vi "main_camera_acquisition.vi"() -> ()   [LabVIEW 2009]
uses:
  <vilib>/userdefined/High Color/IMAQdx.ctl
  <vilib>/vision/Image Controls.llb/IMAQ Image.ctl
  <vilib>/vision/driver/IMAQdx.llb/IMAQdx Buffer Number Mode.ctl
  <vilib>/vision/driver/NI_Vision_Acquisition_Software.lvlib
  Program Files (x86)/National Instruments/LabVIEW 2009/resource/objmgr/imaqdx.rc
panel:
  in  "Video Mode":u32=2
  out "ROI table":string[](array[string])=["Breite [px]", "Höhe [px]", "X-Offset [px]", "Y-Offset [px]"]
  in  "Vollbild":bool
  in  "Y Offset (px)":u32
  in  "X Offset (px)":u32
  in  "Image Height (px)":u32=480
  in  "Image Width (px)":u32=640
  in  "ROI":i32[](array[numeric])=[640, 480, 0, 0]
  in  "Shutter time (ms)":u16(ring)=3 items=["1000", "500", "200", "100", "50", "20", "10", "1"]
  out "Buffer Overrun":bool
  out "Buffer Number":u32
  out "Frame Rate (FPS)":dbl format="%#_3g"
  out "Image Memory":T1
  in  "Buffer Interval":u32=1
  out "Ereignis: FrameDone?":refnum<event-registration>
  out "Camera eingeschaltet":bool
  in  "Kamera ON/OFF":bool
  in  "Stopp":bool
  in  "Detektionskamera":T2="cam0"
  out "Error Out":errorcluster
  out "Image Display":T1(plugin-control)
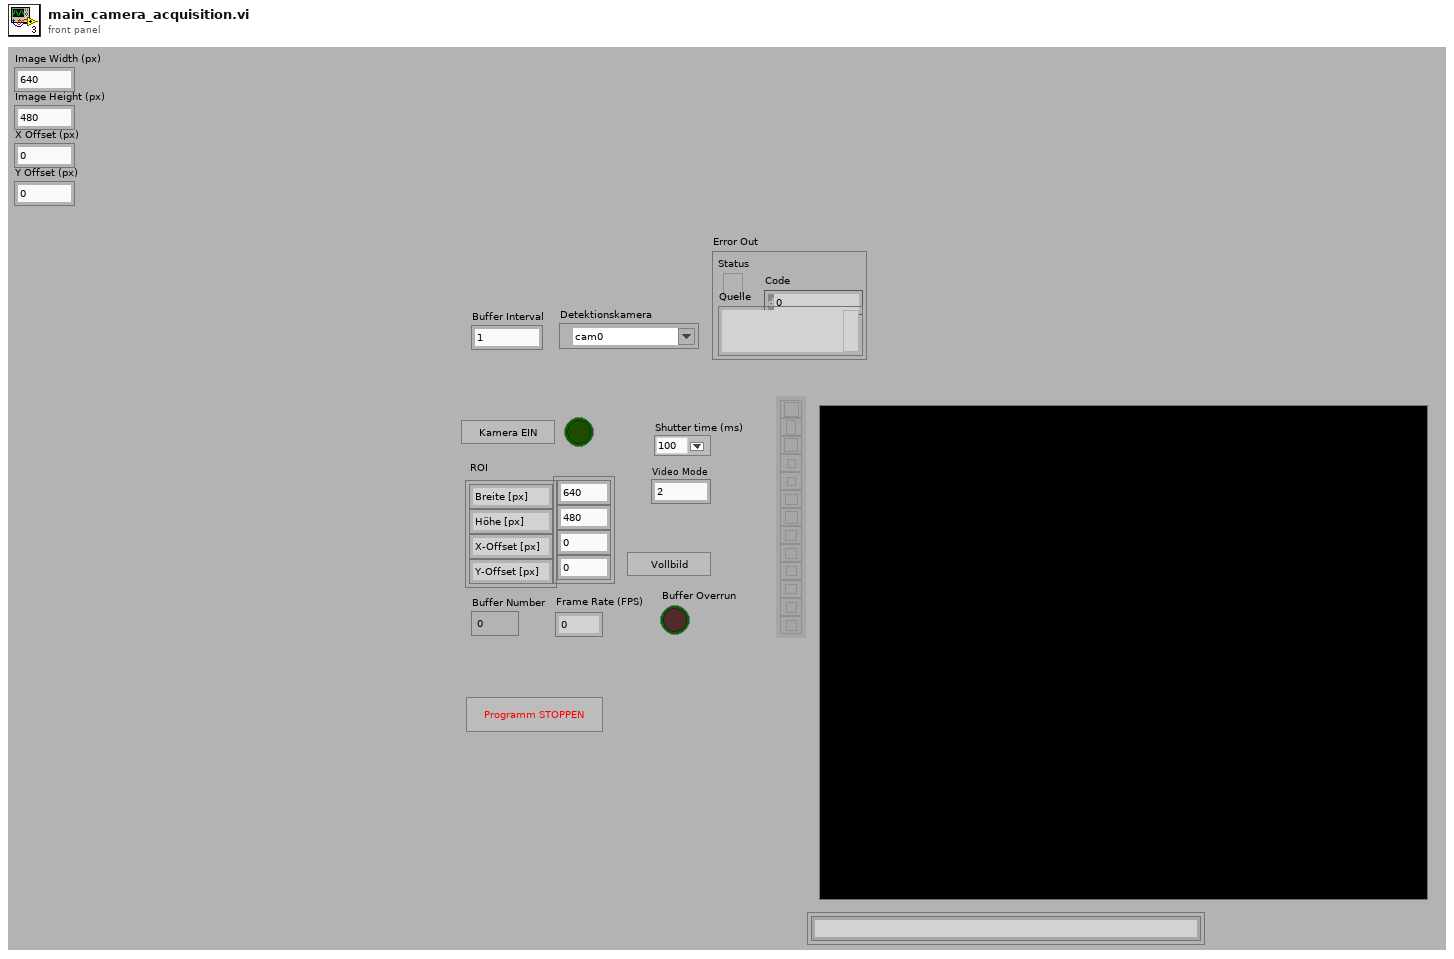
[diagram p1: front panel]
types:
  T1 = typedef "IMAQ Image.ctl" = refnum<image>
  T2 = typedef "IMAQdx.ctl" = refnum<k21>
  T3 = typedef "NI_Vision_Acquisition_Software.lvlib/IMAQdx Buffer Number Mode.ctl" = enum32{"Next", "Last", "Buffer Number"}
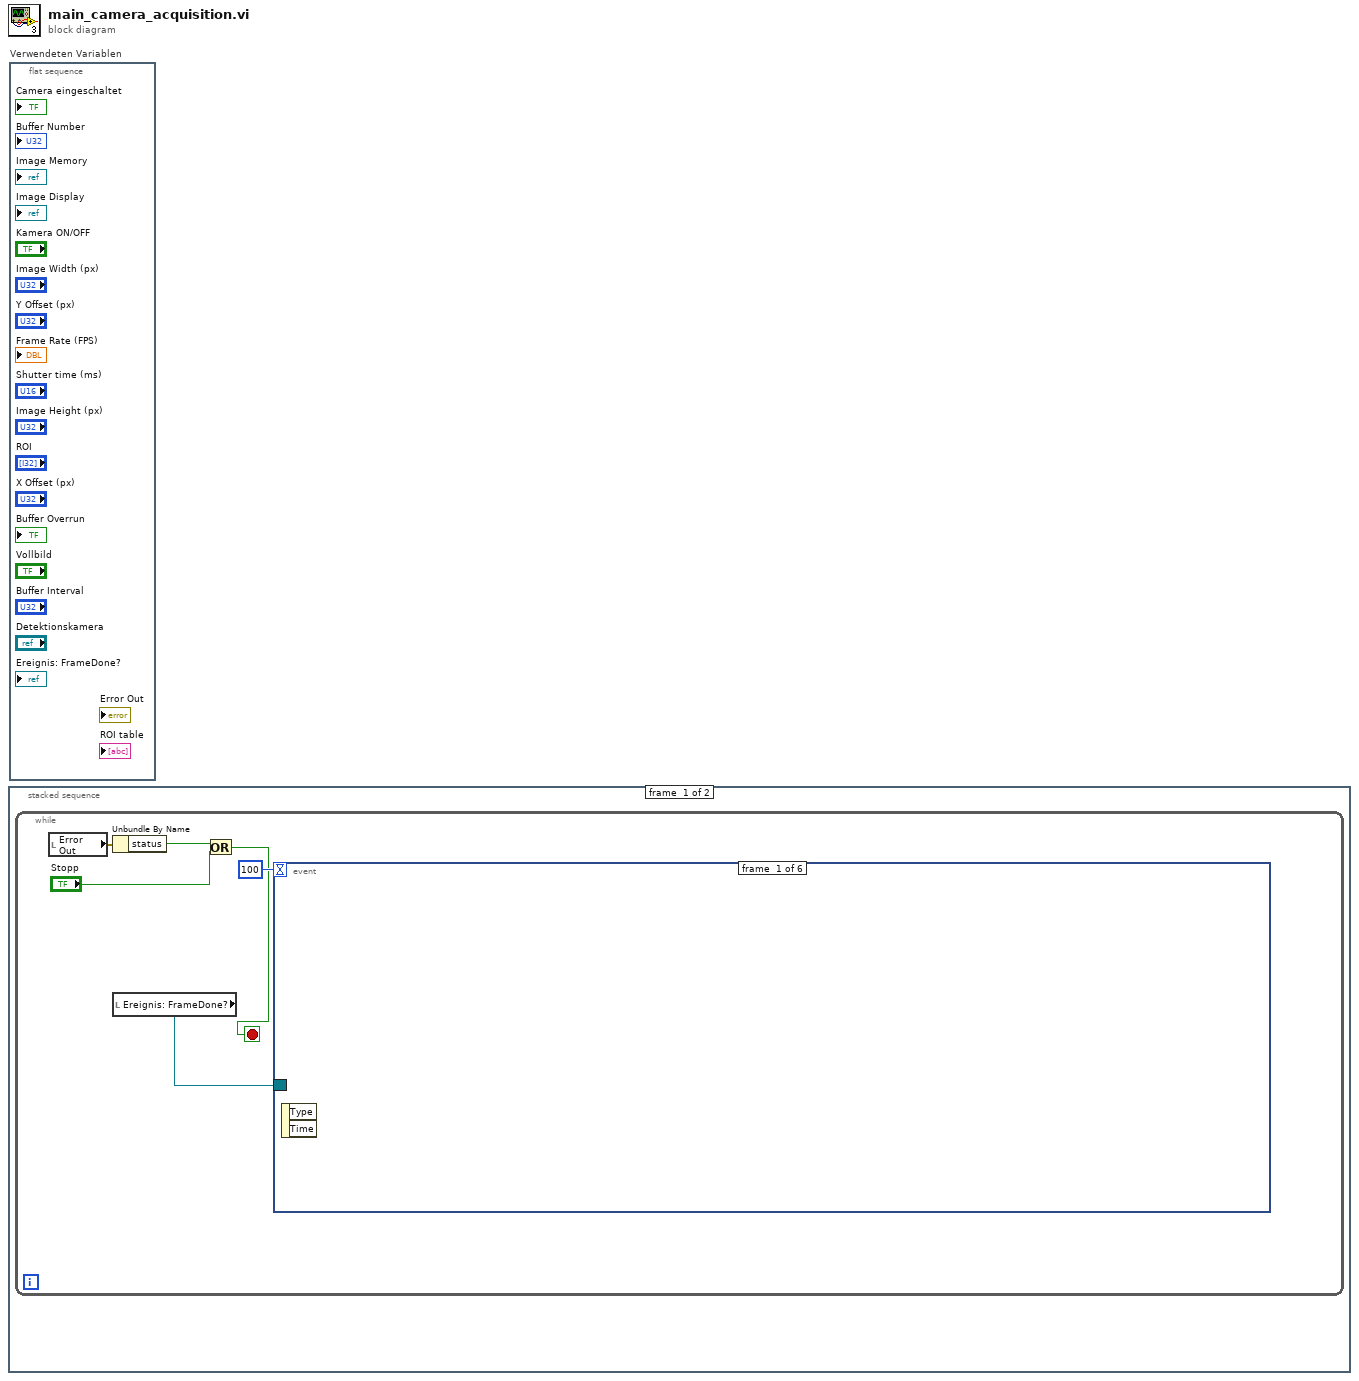
[diagram p0: block diagram]
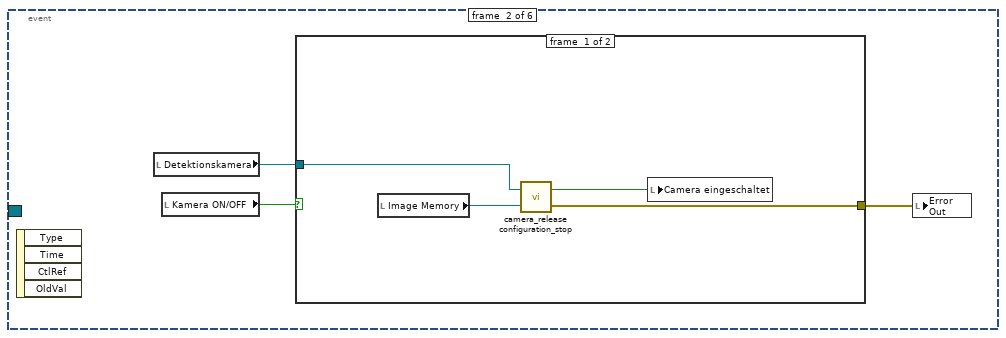
[diagram p2: hidden frame]
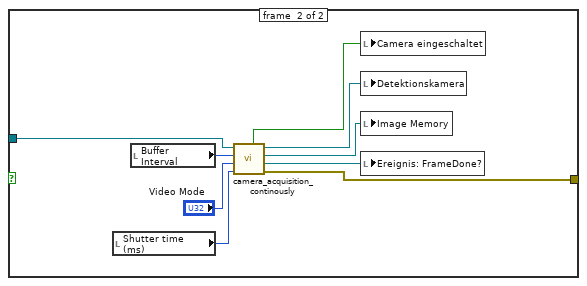
[diagram p3: hidden frame]
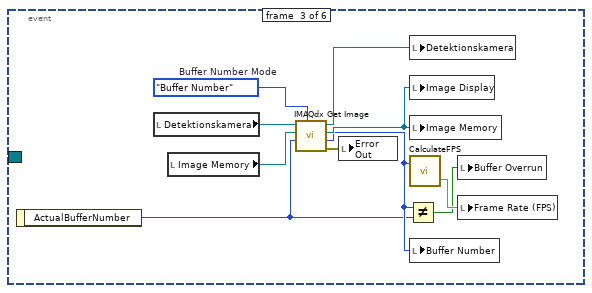
[diagram p4: hidden frame]
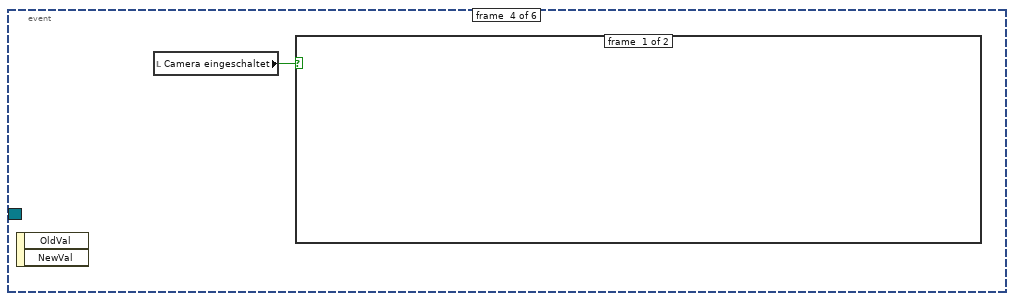
[diagram p5: hidden frame]
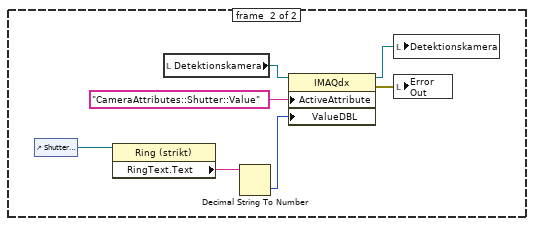
[diagram p6: hidden frame]
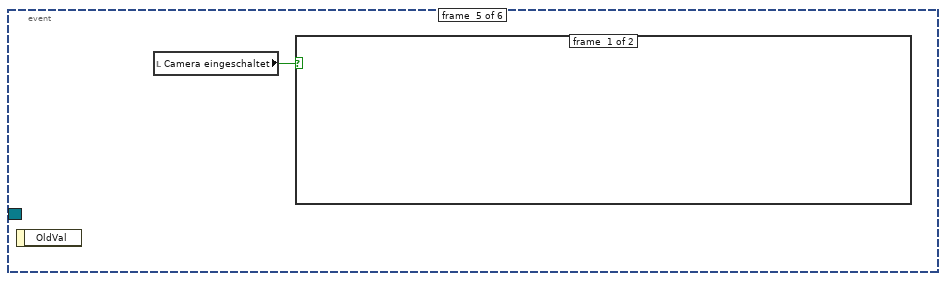
[diagram p7: hidden frame]
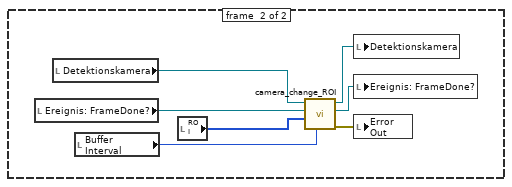
[diagram p8: hidden frame]
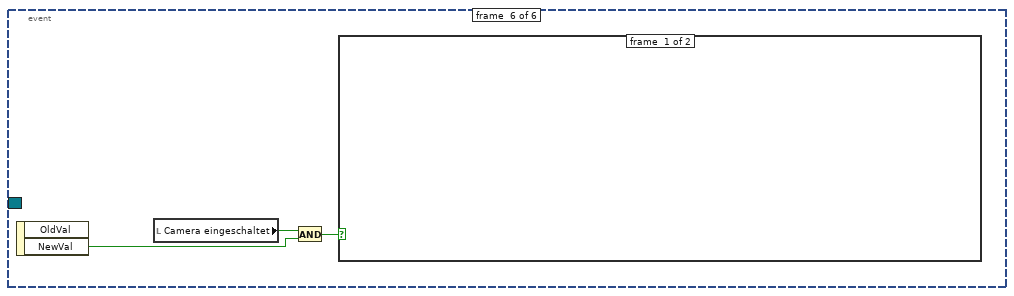
[diagram p9: hidden frame]
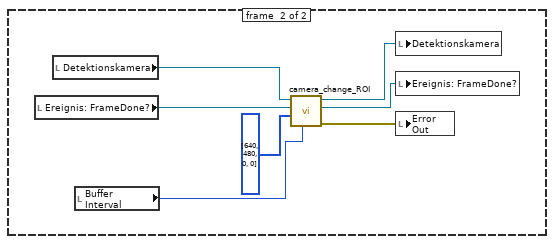
[diagram p10: hidden frame]
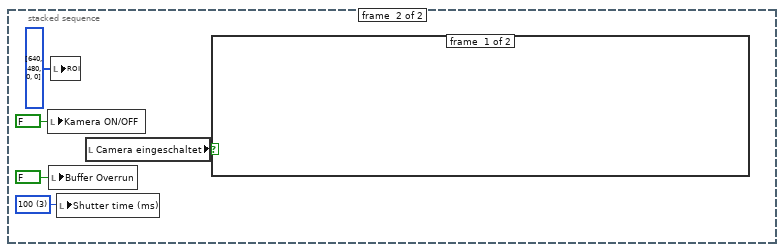
[diagram p11: hidden frame]
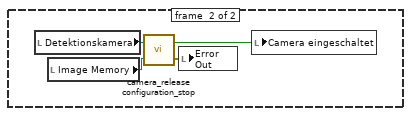
[diagram p12: hidden frame]
diagram:
  n1 = stacked-sequence {
    frame #0 {
      n2 = while {
        stop <- w3 stop-if-true
        n3 = local read "Error Out"() -> (w2:errorcluster)
        n4 = Unbundle By Name(w2) -> ("status"=w1:bool)
        n5 = local read "Ereignis: FrameDone?"() -> (w5:refnum<event-registration>)
        n6 = Or(x=w1, y="Stopp") -> (x .or. y?=w3:bool)
        n7 = event shown="[1] \"Kamera ON/OFF\": Wertänderung" {
          selector: w5 -> [_ _ _ _ _ _]
          dyn-events: _ -> [_ _ _ _ _ _]
          timeout: 100 -> [_ _ _ _ _ _]
          event #0 {
            n8 = event-data() -> ()  [unwired: 1 in, 2 out]
          }
          event #1 {
            n9 = event-data() -> ()  [unwired: 1 in, 4 out]
            n10 = local read "Detektionskamera"() -> (w8:T2)
            n11 = local read "Kamera ON/OFF"() -> (w9:bool)
            n12 = case shown="True" w9 {
              tunnel: w8 -> [w10 w17]
              tunnel: [w13 w18] -> w7
              frame #0 {
                n13 = local read "Image Memory"() -> (w11:T1)
                n14 = call "camera_release configuration_stop.vi"("Image Memory"=w11, "Detektionskamera"=w10) -> ("error out"=w13:errorcluster, "status"=w12:bool)
                n15 = local write "Camera eingeschaltet"(w12) -> ()
              }
              frame #1 {
                n16 = local read "Shutter time (ms)"() -> (w14:u16)
                n17 = local read "Buffer Interval"() -> (w16:u32)
                n18 = call "camera_acquisition_continously.vi"("Detektionskamera"=w17, "BufferInterval"=w16, "Video Mode"="Video Mode", "Shutter time (ms)"=w14) -> ("Kamera eingeschaltet?"=w22:bool, "Detektionskamera"=w21:T2, "Image Memory"=w20:T1, "Ereignis: FrameDone?"=w19:refnum<event-registration>, "error out"=w18:errorcluster)
                n19 = local write "Camera eingeschaltet"(w22) -> ()
                n20 = local write "Detektionskamera"(w21) -> ()
                n21 = local write "Image Memory"(w20) -> ()
                n22 = local write "Ereignis: FrameDone?"(w19) -> ()
              }
            }
            n23 = local write "Error Out"(w7) -> ()
          }
          event #2 {
            w32 = IMAQdx_Buffer_Number_Mode."Buffer Number"  # Buffer Number Mode
            n24 = event-data() -> ("ActualBufferNumber"=w24:u32)  [unwired: 1 in]
            n25 = local read "Detektionskamera"() -> (w30:T2)
            n26 = local read "Image Memory"() -> (w29:T1)
            n27 = call <vilib>:"IMAQdx Get Image.vi"("Buffer Number Mode (Next)"=w32, "Buffer Number In"=w24, "Image In"=w29, "Session In"=w30) -> ("error out"=w31:errorcluster, "Buffer Number Out"=w25:u32, "Image Out"=w27:T1, "Session Out"=w26:T2)  [unwired: 1 in, 3 out]
            n28 = local write "Error Out"(w31) -> ()
            n29 = Not Equal?(x=w25, y=w24) -> (x != y?=w23:bool)
            n30 = local write "Detektionskamera"(w26) -> ()
            n31 = local write "Image Display"(w27) -> ()
            n32 = local write "Image Memory"(w27) -> ()
            n33 = call "CalculateFPS.vi"("buffer number"=w25) -> ("processed FPS"=w28:dbl)  [unwired: 2 out]
            n34 = local write "Buffer Number"(w25) -> ()
            n35 = local write "Buffer Overrun"(w23) -> ()
            n36 = local write "Frame Rate (FPS)"(w28) -> ()
          }
          event #3 {
            n37 = event-data() -> ()  [unwired: 1 in, 2 out]
            n38 = local read "Camera eingeschaltet"() -> (w33:bool)
            n39 = case shown="True" w33 {
              frame #0 {
              }
              frame #1 {
                n40 = control-ref of="Shutter time (ms)"() -> (w40:refnum<vi>)
                n41 = property class="Ring (strikt)"(reference=w40) -> ("RingText.Text"=w39:string)  [unwired: 1 in, 2 out]
                n42 = local read "Detektionskamera"() -> (w38:T2)
                n43 = Decimal String To Number(string=w39) -> (number=w34:i32)  [unwired: 2 in, 1 out]
                n44 = property class="IMAQdx"(reference=w38, "ActiveAttribute"="CameraAttributes::Shutter::Value", "ValueDBL"=w34) -> (reference out=w37:T2, error out=w36:errorcluster)  [unwired: 1 in]
                n45 = local write "Detektionskamera"(w37) -> ()
                n46 = local write "Error Out"(w36) -> ()
              }
            }
          }
          event #4 {
            n47 = event-data() -> ()  [unwired: 1 in, 1 out]
            n48 = local read "Camera eingeschaltet"() -> (w41:bool)
            n49 = case shown="True" w41 {
              frame #0 {
              }
              frame #1 {
                n50 = local read "Ereignis: FrameDone?"() -> (w42:refnum<event-registration>)
                n51 = local read "Detektionskamera"() -> (w47:T2)
                n52 = local read "Buffer Interval"() -> (w46:u32)
                n53 = local read "ROI"() -> (w48:i32[])
                n54 = call "camera_change_ROI.vi"("BufferInterval"=w46, "Region of Interest"=w48, "Ereignisregistrierung (Referenz) 2"=w42, "Session In"=w47) -> ("Fehler (Ausgang)"=w44:errorcluster, "Ereignisregistrierung (Referenz)"=w45:refnum<event-registration>, "Session Out"=w43:T2)  [unwired: 5 in]
                n55 = local write "Detektionskamera"(w43) -> ()
                n56 = local write "Ereignis: FrameDone?"(w45) -> ()
                n57 = local write "Error Out"(w44) -> ()
              }
            }
          }
          event #5 {
            n58 = event-data() -> ("NewVal"=w50:bool)  [unwired: 1 in, 1 out]
            n59 = local read "Camera eingeschaltet"() -> (w51:bool)
            n60 = And(x=w51, y=w50) -> (x .and. y?=w49:bool)
            n61 = case shown="True" w49 {
              frame #0 {
              }
              frame #1 {
                n62 = local read "Ereignis: FrameDone?"() -> (w53:refnum<event-registration>)
                n63 = local read "Detektionskamera"() -> (w58:T2)
                n64 = local read "Buffer Interval"() -> (w57:u32)
                n65 = call "camera_change_ROI.vi"("BufferInterval"=w57, "Region of Interest"=i32[] [640, 480, 0, 0] ("Region of Interest (px)"), "Ereignisregistrierung (Referenz) 2"=w53, "Session In"=w58) -> ("Fehler (Ausgang)"=w55:errorcluster, "Ereignisregistrierung (Referenz)"=w56:refnum<event-registration>, "Session Out"=w54:T2)  [unwired: 5 in]
                n66 = local write "Detektionskamera"(w54) -> ()
                n67 = local write "Ereignis: FrameDone?"(w56) -> ()
                n68 = local write "Error Out"(w55) -> ()
              }
            }
          }
        }
      }
    }
    frame #1 {
      w60 = u16 3 items=["1000", "500", "200", "100", "50", "20", "10"] ("Shutter time (ms)")
      n69 = local write "Kamera ON/OFF"(FALSE ("Kamera ON/OFF")) -> ()
      n70 = local write "Buffer Overrun"(FALSE ("Kamera ON/OFF")) -> ()
      n71 = local write "ROI"(i32[] [640, 480, 0, 0] ("Region of Interest (px)")) -> ()
      n72 = local write "Shutter time (ms)"(w60) -> ()
      n73 = local read "Camera eingeschaltet"() -> (w63:bool)
      n74 = case shown="True" w63 {
        frame #0 {
        }
        frame #1 {
          n75 = local read "Detektionskamera"() -> (w64:T2)
          n76 = local read "Image Memory"() -> (w67:T1)
          n77 = call "camera_release configuration_stop.vi"("Image Memory"=w67, "Detektionskamera"=w64) -> ("error out"=w65:errorcluster, "status"=w66:bool)
          n78 = local write "Error Out"(w65) -> ()
          n79 = local write "Camera eingeschaltet"(w66) -> ()
        }
      }
    }
  }
  n80 = flat-sequence "Verwendeten Variablen" {
    frame #0 {
    }
  }
